vi "Set Log File And Paths.vi"(6 "timeout (ms)":i32=-1, 8 "error in (no error)":errorcluster, 9 "File Path":string, 10 "File Name":string, 11 "FlexLogger_gRPCAPI in":refnum<class "FlexLogger_gRPC.lvclass">) -> (0 "error out":errorcluster, 3 "FlexLogger_gRPCAPI out":refnum<class "FlexLogger_gRPC.lvclass">)   [LabVIEW 2020, in "FlexLogger_gRPC.lvlib" / "FlexLogger_gRPC.lvclass"]
uses:
  FlexLogger_gRPC.lvclass
  FlexLogger_client/RPC Messages/flexlogger_SetLogFileNameRequest.ctl
  FlexLogger_client/RPC Messages/flexlogger_ElementIdentifier.ctl
  FlexLogger_client/RPC Messages/flexlogger_SetLogFileBasePathRequest.ctl
  FlexLogger_gRPC.lvclass/FlexLogger_gRPC.ctl
  FlexLogger_client/FlexLogger_client.lvlib
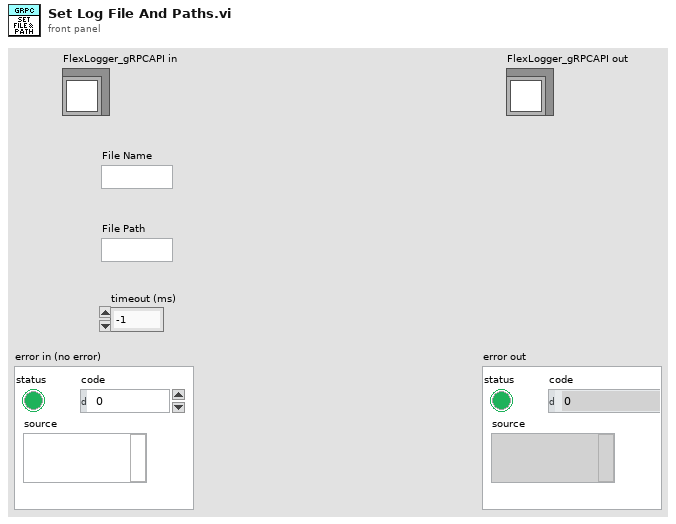
[diagram p1: front panel]
types:
  T1 = typedef "FlexLogger_client.lvlib/flexlogger_SetLogFileBasePathRequest.ctl" = cluster{"document_identifier":T2, "log_file_base_path":string}
  T2 = typedef "FlexLogger_client.lvlib/flexlogger_ElementIdentifier.ctl" = cluster{"project_id":string, "file_name":string, "element_id":string, "subpart_id":string}
  T3 = typedef "FlexLogger_client.lvlib/flexlogger_SetLogFileNameRequest.ctl" = cluster{"document_identifier":T2, "log_file_name":string}
  T4 = typedef "grpc-lvsupport-release.lvlib/grpcId.ctl" = u64
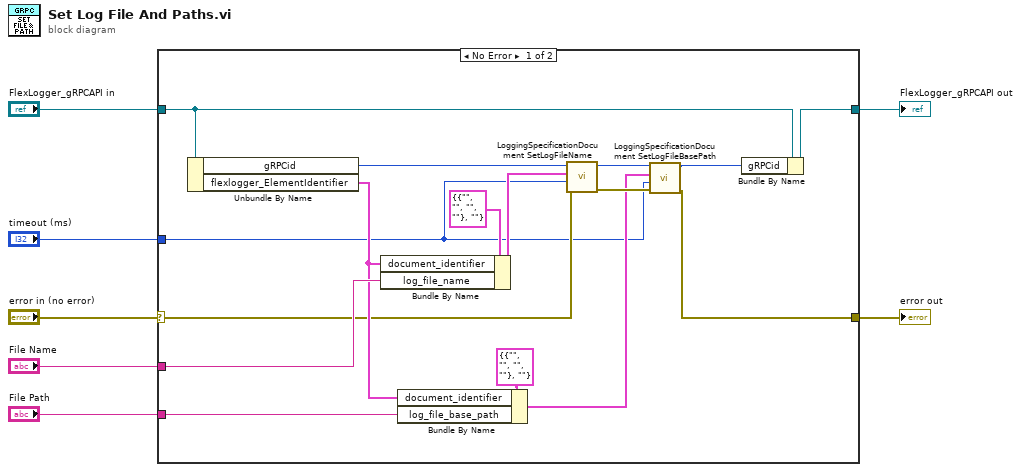
[diagram p0: block diagram]
diagram:
  n1 = case shown="No Error" "error in (no error)" {
    selector: "error in (no error)" -> [w9 w24]
    tunnel: "FlexLogger_gRPCAPI in" -> [w23 w25]
    tunnel: [w22 w25] -> w7
    tunnel: [w19 w24] -> w5
    tunnel: "File Name" -> [w16 _]
    tunnel: "File Path" -> [w14 _]
    tunnel: "timeout (ms)" -> [w8 _]
    frame No Error {
      n2 = Unbundle By Name(w23) -> ("gRPCid"=w11:T4, "flexlogger_ElementIdentifier"=w10:T2)
      n3 = Bundle By Name(cluster=T3 {"document_identifier"={"project_id"="", "file_name"="", "element_id"="", "subpart_id"=""}, "log_file_name"=""} ("Request Data"), "document_identifier"=w10, "log_file_name"=w16) -> (w15:T3)
      n4 = Bundle By Name(cluster=T1 {"document_identifier"={"project_id"="", "file_name"="", "element_id"="", "subpart_id"=""}, "log_file_base_path"=""} ("Request Data"), "document_identifier"=w10, "log_file_base_path"=w14) -> (w13:T1)
      n5 = call "LoggingSpecificationDocument SetLogFileName.vi"("error in"=w9, "timeout (ms)"=w8, "Request Data"=w15, "gRPC ID"=w11) -> ("error out"=w20:errorcluster, "gRPC ID out"=w21:T4)  [unwired: 5 in, 1 out]
      n6 = call "LoggingSpecificationDocument SetLogFileBasePath.vi"("error in"=w20, "timeout (ms)"=w8, "Request Data"=w13, "gRPC ID"=w21) -> ("error out"=w19:errorcluster, "gRPC ID out"=w18:T4)  [unwired: 5 in, 1 out]
      n7 = Bundle By Name(cluster=w23, "gRPCid"=w18) -> (w22:refnum<class "FlexLogger_gRPC.lvclass">)
    }
    frame Error {
    }
  }
  "error out" <- w5
  "FlexLogger_gRPCAPI out" <- w7
